vi "setup_sub.vi"(4 "OutputPinMsk":u16 format="%x", 5 "servoEnableMask":u8, 6 "ENC_RES_Array":u16[](array[numeric]), 7 "motorEnableMask":u8, 8 "pinLocation_Array":u8[](array[numeric]), 9 "Loop Frequency":u16=10000 min=1, 10 "ADC_Settings":u16[](array[ring]) items=["Range_CH_OFF_msk"=0, "Range_pm_10_24_msk"=1, "Range_pm_05_12_msk"=2, "Range_pm_02_56_msk"=3, "Range_pm_01_28_msk"=4, "Range_pm_00_64_msk"=5, "Range_10_24_msk"=9, "Range_05_12_msk"=10, "Range_02_56_msk"=11, "Range_01_28_msk"=12, "Range_00_64_msk"=13], 11 "instance":i32) -> (3 "Success?":bool)   [LabVIEW 2025]
uses:
  LVLib/SADI_FW3.lvlib
panel:
  out "result":u32
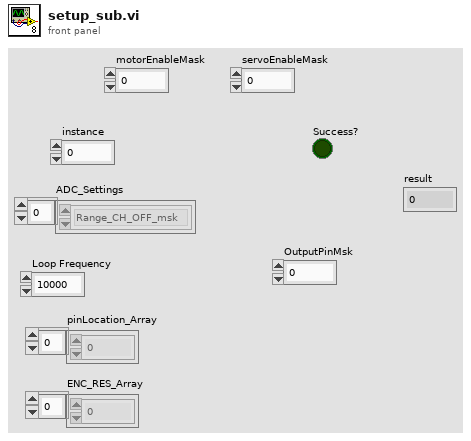
[diagram p1: front panel]
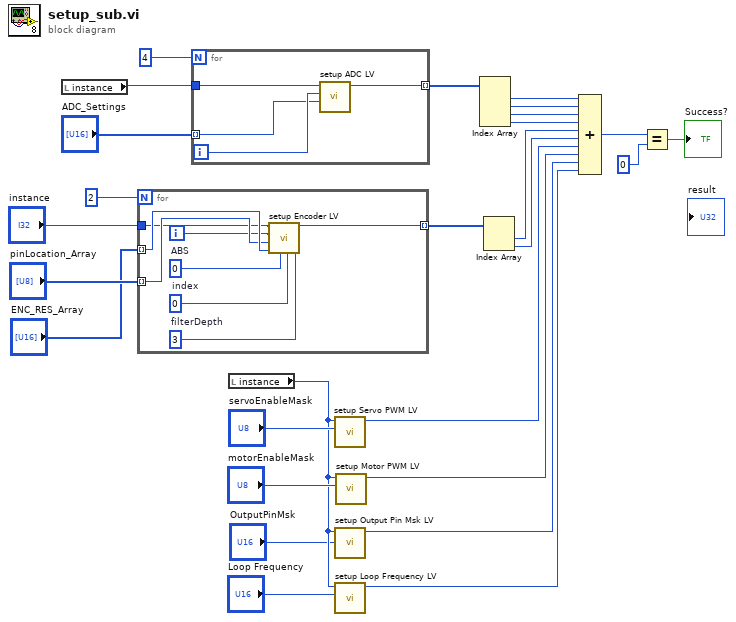
[diagram p0: block diagram]
diagram:
  n1 = local read "instance"() -> (w23:i32)
  n2 = for {
    N: 2 -> [_]
    tunnel: "instance" -> [w29]
    tunnel: "pinLocation_Array" -> [w31] mode=indexing
    tunnel: "ENC_RES_Array" -> [w32] mode=indexing
    tunnel: [w28] -> w4 mode=indexing
    i -> [w30]
    w34 = u8 0  # index
    w33 = u8 3  # filterDepth
    w35 = u8 0  # ABS
    n3 = call "setup Encoder LV.vi"("filterDepth"=w33, "index"=w34, "ABS"=w35, "resolution"=w32, "pinLocation"=w31, "encoderNum"=w30, "instance"=w29) -> ("function return"=w28:u32)  [unwired: 4 in]
  }
  n4 = for {
    N: 4 ("Numeric") -> [_]
    tunnel: "ADC_Settings" -> [w38] mode=indexing
    tunnel: w23 -> [w37]
    tunnel: [w36] -> w16 mode=indexing
    i -> [w39]
    n5 = call "setup ADC LV.vi"("adcSetting"=w38, "adcNum"=w39, "instance"=w37) -> ("function return"=w36:u32)  [unwired: 8 in]
  }
  n6 = local read "instance"() -> (w17:i32)
  n7 = call "setup Servo PWM LV.vi"("servoEnables"="servoEnableMask", "instance"=w17) -> ("function return"=w1:u32)  [unwired: 9 in]
  n8 = call "setup Output Pin Msk LV.vi"("OutputPinMsk"="OutputPinMsk", "instance"=w17) -> ("function return"=w2:u32)  [unwired: 9 in]
  n9 = call "setup Loop Frequency LV.vi"("frequency"="Loop Frequency", "instance"=w17) -> ("function return"=w6:u32)  [unwired: 9 in]
  n10 = call "setup Motor PWM LV.vi"("motorEnables"="motorEnableMask", "instance"=w17) -> ("function return"=w3:u32)  [unwired: 9 in]
  n11 = Index Array(array=w16) -> (element #1=w7:u32, element #2=w15:u32, element #3=w9:u32, element #4=w8:u32)  [unwired: 4 in]
  n12 = Index Array(array=w4) -> (element #1=w10:u32, element #2=w5:u32)  [unwired: 2 in]
  n13 = Compound Arithmetic op=ADD(w7, w15, w9, w8, w10, w5, w1, w3, w2, w6) -> (w14:u32)
  n14 = Equal?(x=w14, y=u32 0) -> (x = y?=→"Success?":bool)
